vi "BinanceAPI_START_BINANCE.vi"(0 "API KEY":string, 5 "Secred API":string, 11 "error in (no error)":errorcluster) -> (4 "BinanceAPI":refnum<class "BinanceAPI_.lvclass">, 14 "All is OK? (True = OK)":bool, 15 "error out":errorcluster)   [LabVIEW 2022 SP3, in "BinanceAPI_.lvclass"]
doc: "Initialize BinanceAPI. <B>Must be always used</B> on the begining of the BinanceAPI class chain\n\nFirst generate API key's:\n\nAPI Key Setup\n\n Some endpoints will require an API Key. Regarding API key creation, please refer to:\n - <B>https://www.binancezh.top/en/support/faq/360002502072</B> .\n Once API key is created, it is recommended to set IP restrictions on the key for security rseasons.\n Never share your API key/secret key to <B>ANYONE</B>.\n\nIf the API keys were accidentally shared, please delete them immediately and create a new key.\n\nAPI Key Restrictions\n\n After creating the API key, the default restrictions is Enable Reading.\n To enable withdrawals via the API, the API key restriction needs to be modified through the Binance UI and You should contact with autor of BinanceAPI (there is no open source files enable to automatic withdraws)."
uses:
  BinanceAPI_.lvclass
  BinanceAPI_.lvclass/BinanceAPI_.ctl
  <vilib>/httpClient/LabVIEWHTTPClient.lvlib
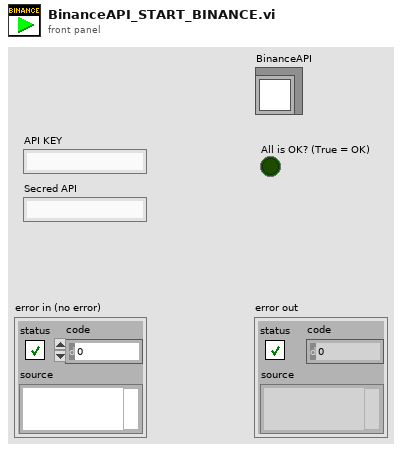
[diagram p1: front panel]
types:
  T1 = typedef "LabVIEWHTTPClient.lvlib/ClientHandle.ctl" = refnum<k1>
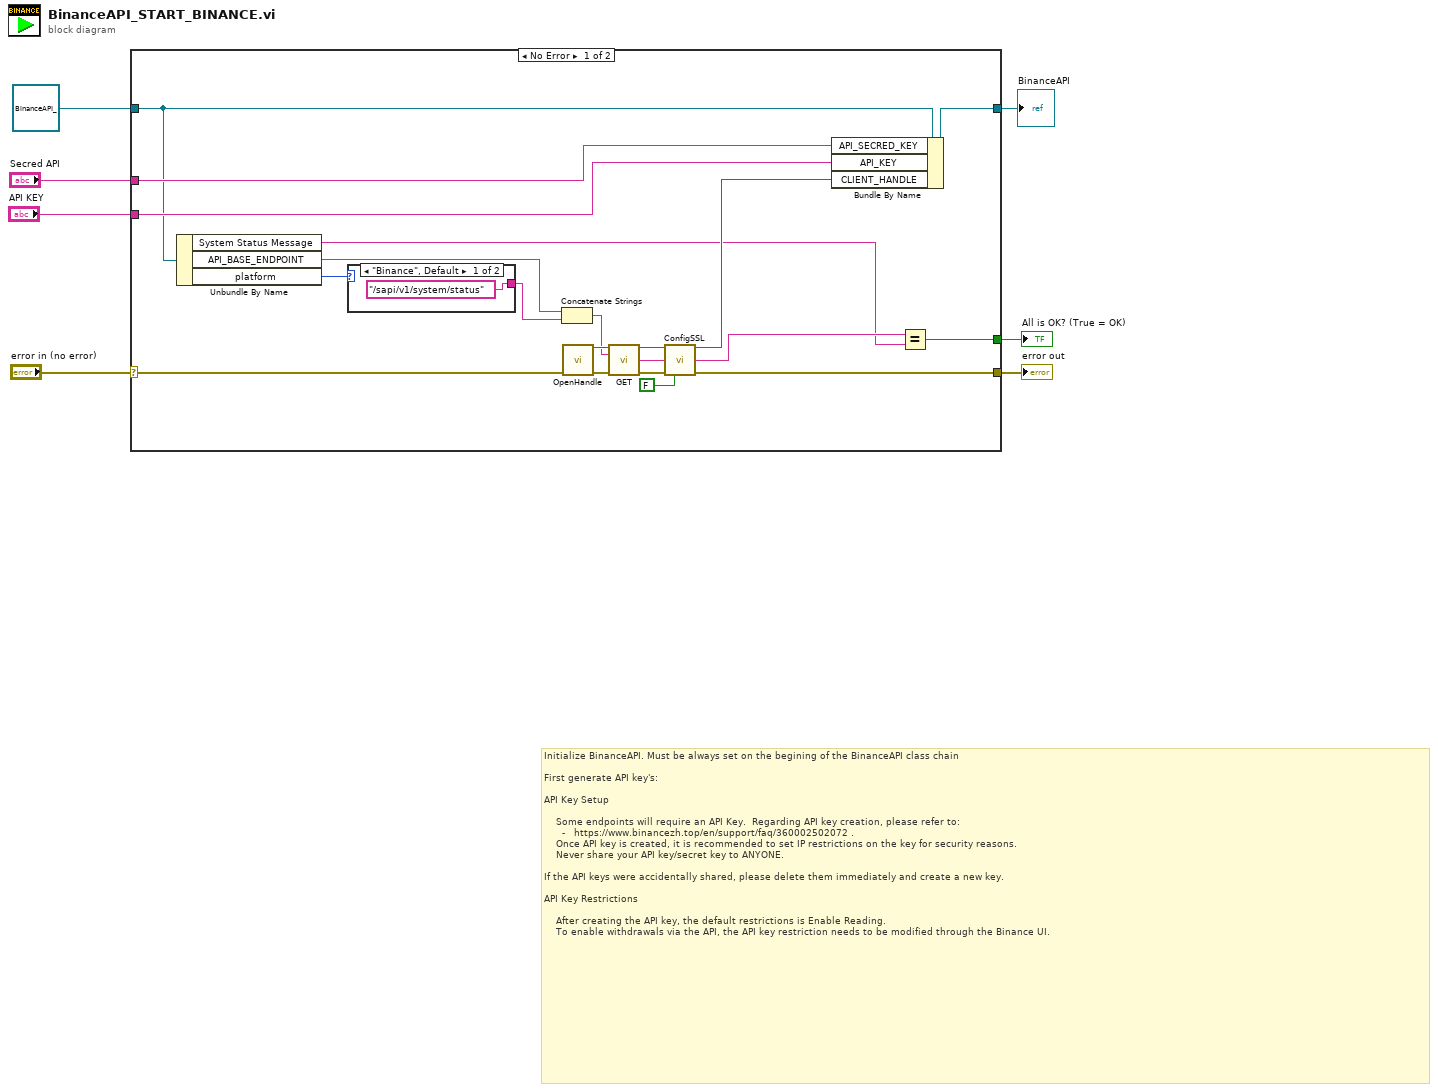
[diagram p0: block diagram]
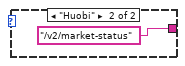
[diagram p2: hidden frame]
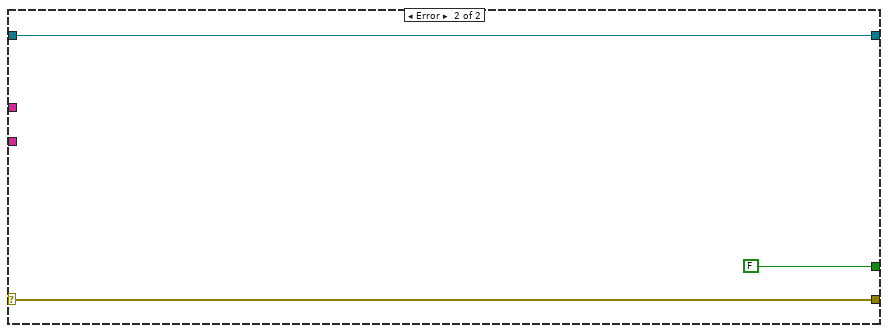
[diagram p3: hidden frame]
diagram:
  # "Initialize BinanceAPI. Must be always set on the begining of the BinanceAPI class chain\n\nFirst generate API key's:\n\nAPI Key Setup\n\n    Some endpoints will require an API Key.  Regarding API key creation, please refer to:\n      -   https://www.binancezh.top/en/support/faq/360002502072 .\n    Once API key is created, it is recommended to set IP restrictions on the key for security reasons.\n    Never share your API key/secret key to ANYONE.\n\nIf the API keys were accidentally shared, please delete them immediately and create a new key.\n\nAPI Key Restrictions\n\n    After creating the API key, the default restrictions is Enable Reading.\n    To enable withdrawals via the API, the API key restriction needs to be modified through the Binance UI."
  n1 = case shown="No Error" "error in (no error)" {
    selector: "error in (no error)" -> [w25 w31]
    tunnel: [w10 w31] -> w6
    tunnel: [w26 w30] -> w2
    tunnel: refnum<class "BinanceAPI_.lvclass"> refnum ("BinanceAPI_.lvclass") -> [w16 w30]
    tunnel: "API KEY" -> [w22 _]
    tunnel: "Secred API" -> [w21 _]
    tunnel: [w17 FALSE] -> w3
    frame No Error {
      n2 = Unbundle By Name(w16) -> ("System Status Message"=w9:string, "API_BASE_ENDPOINT"=w15:string, "platform"=w8:enum16{"Binance", "Huobi", "Coinbase"})
      n3 = case shown="\"Binance\", Default" w8 {
        tunnel: ["/sapi/v1/system/status" "/v2/market-status"] -> w20
        frame "Binance", Default {
        }
        frame "Huobi" {
        }
      }
      n4 = Concatenate Strings(w15, w20) -> (w19:string)
      n5 = call <vilib>:"OpenHandle.vi"("error in (no error)"=w25) -> ("client handle out"=w23:T1, "error out"=w24:errorcluster)  [unwired: 13 in]
      n6 = call <vilib>:"GET.vi"("client handle"=w23, "url"=w19, "error in (no error)"=w24) -> ("client handle out"=w13:T1, "body"=w18:string, "error out"=w11:errorcluster)  [unwired: 9 in, 1 out]
      n7 = call <vilib>:"ConfigSSL.vi"("client handle"=w13, "error in (no error)"=w11, "verify server (true)"=FALSE) -> ("client handle out"=w12:T1, "error out"=w10:errorcluster)  [unwired: 11 in]
      n8 = Bundle By Name(cluster=w16, "API_SECRED_KEY"=w21, "API_KEY"=w22, "CLIENT_HANDLE"=w12) -> (w26:refnum<class "BinanceAPI_.lvclass">)
      n9 = Equal?(x=w18, y=w9) -> (x = y?=w17:bool)
    }
    frame Error {
    }
  }
  "error out" <- w6
  "All is OK? (True = OK)" <- w3
  "BinanceAPI" <- w2
